vi "Logger_Destroy.vi"(8 "error in (no error)":errorcluster caption="错误输入（无错误）", 11 "Logger 输入":refnum<class "Logger.lvclass">) -> (0 "error out":errorcluster caption="错误输出", 3 "Logger 输出":refnum<class "Logger.lvclass">)   [LabVIEW 2019, in "Logger.lvclass"]
uses:
  <userlib>/Logger/Logger.lvclass
  <userlib>/Logger/Logger.lvclass/Logger.ctl
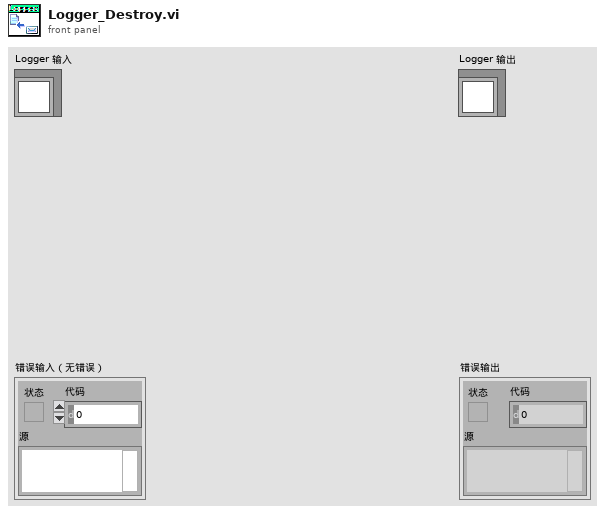
[diagram p1: front panel]
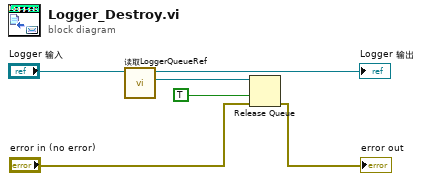
[diagram p0: block diagram]
diagram:
  n1 = call "读取LoggerQueueRef.vi"("Logger输入"="Logger 输入") -> ("LoggerQueueRef"=w3:refnum<queue>, "Logger输出"=→"Logger 输出":refnum<class "Logger.lvclass">)  [unwired: 8 in, 1 out]
  n2 = Release Queue(queue=w3, force destroy? (F)=TRUE ("强制销毁？(F)"), error in (no error)="error in (no error)") -> (error out=→"error out":errorcluster)  [unwired: 2 out]
